vi "Type_Bench.vi"(8 "error in (no error)":errorcluster caption="entrée d'erreur (pas d'erreur)", 10 "Bench Type":T1, 11 "Class Instrument Firebase Altyor en entrée":refnum<class "Class Instrument Firebase Altyor.lvclass">) -> (0 "error out":errorcluster caption="sortie d'erreur", 3 "Class Instrument Firebase Altyor en sortie":refnum<class "Class Instrument Firebase Altyor.lvclass">)   [LabVIEW 2020, in "Library Instrument & Equipement.lvlib" / "Library Instruments.lvlib" / "Class Instrument Firebase Altyor.lvclass"]
uses:
  Class Instrument Firebase Altyor.lvclass
  Commun VI/TypeDef/Bench Type.ctl
  Class Instrument Firebase Altyor.lvclass/Class Instrument Firebase Altyor.ctl
  Commun VI/Library Commun.lvlib
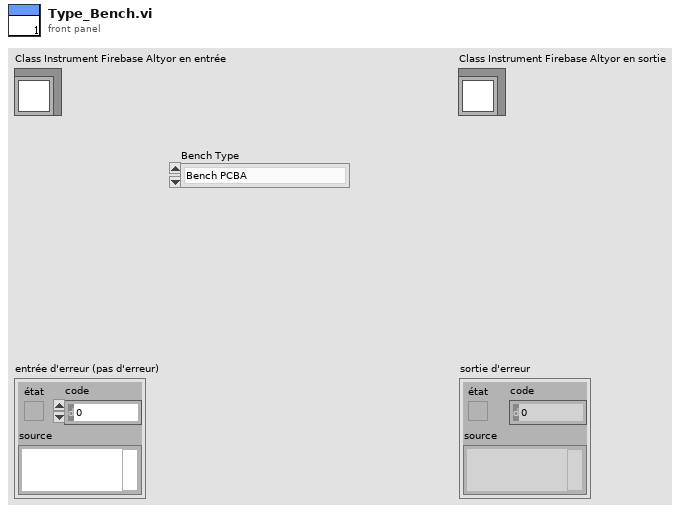
[diagram p1: front panel]
types:
  T1 = typedef "Library Commun.lvlib/Bench Type.ctl" = enum16{"Bench PCBA", "Bench Camera", "Bench Assembly", "Bench PCBA P2193"}
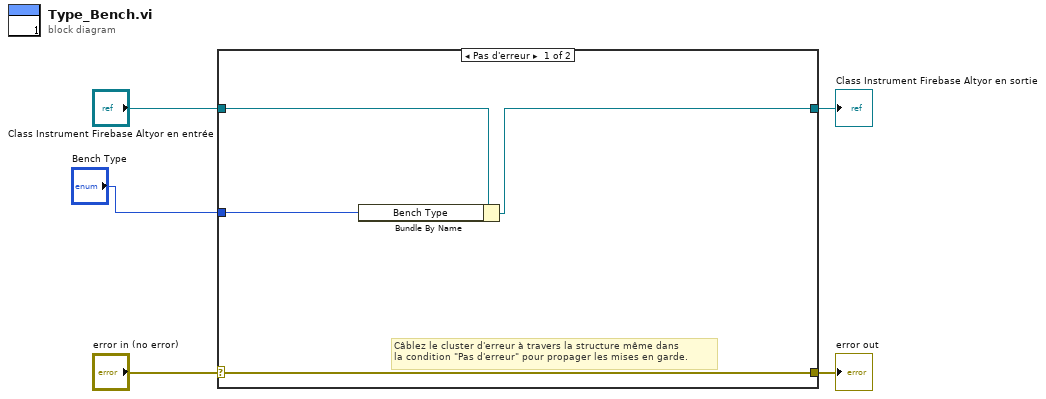
[diagram p0: block diagram]
diagram:
  n1 = case shown="Pas d'erreur" "error in (no error)" {
    selector: "error in (no error)" -> [w9 w11]
    tunnel: [w9 w11] -> w4
    tunnel: [w6 w10] -> w2
    tunnel: "Class Instrument Firebase Altyor en entrée" -> [w7 w10]
    tunnel: "Bench Type" -> [w8 _]
    frame No Error {
      # "Câblez le cluster d'erreur à travers la structure même dans\nla condition \"Pas d'erreur\" pour propager les mises en garde."
      n2 = Bundle By Name(cluster=w7, "Bench Type"=w8) -> (w6:refnum<class "Class Instrument Firebase Altyor.lvclass">)
    }
    frame Error {
    }
  }
  "error out" <- w4
  "Class Instrument Firebase Altyor en sortie" <- w2
